vi "MV3D RGBD Get Device Number.vi"(10 "pDeviceNumber":u32, 11 "nDeviceType":u32) -> (2 "pDeviceNumber out":u32, 3 "function return":i32)   [LabVIEW 2015, in "Mv3dRgbd.lvlib"]
doc: "MV3D_RGBD_API MV3D_RGBD_STATUS MV3D_RGBD_GetDeviceNumber(uint32_t nDeviceType, uint32_t* pDeviceNumber);"
uses:
  <userlib>/Mv3dRgbd/Mv3dRgbd.lvlib
  <userlib>/Mv3dRgbd/Mv3dRgbd.dll
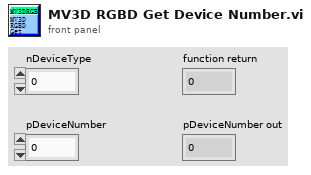
[diagram p1: front panel]
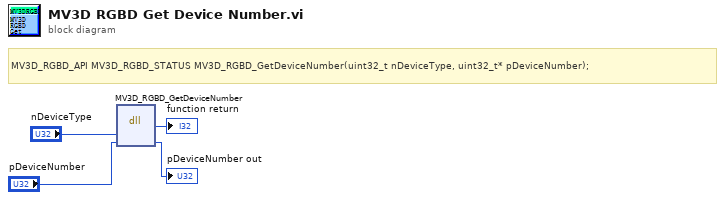
[diagram p0: block diagram]
diagram:
  # "MV3D_RGBD_API MV3D_RGBD_STATUS MV3D_RGBD_GetDeviceNumber(uint32_t nDeviceType, uint32_t* pDeviceNumber);"
  n1 = dll-call lib="C:/Program Files (x86)/National Instruments/LabVIEW 2015/user.lib/Mv3dRgbd/Mv3dRgbd.*" fn="MV3D_RGBD_GetDeviceNumber"("nDeviceType"="nDeviceType", "pDeviceNumber"="pDeviceNumber") -> (→"function return":i32, "pDeviceNumber"=→"pDeviceNumber out":u32)  [unwired: 4 in, 2 out]
